vi "Read XML_Parse BC Major Frames.vi"(8 "error in (no error)":errorcluster, 10 "channel in":T1, 11 ".NET Refnum in":refnum<k24>) -> (0 "error out":errorcluster, 2 "channel out":T1, 3 ".NET Refnum out":refnum<k24>)   [LabVIEW 2017, in "Ballard 1553 System Explorer.lvlib"]
uses:
  Ballard 1553 System Explorer.lvlib
  Ballard_Channel.ctl
  Ballard_BC.ctl
  Ballard_message.ctl
  Ballard_messageType.ctl
  Ballard_CWD1.ctl
  Ballard_CWD2.ctl
  Ballard_minorFrame.ctl
  Ballard_majorFrame.ctl
  Ballard_acyclicFrame.ctl
  Ballard_RT.ctl
  Ballard_RT subAddress.ctl
  Ballard_RT direction.ctl
  Ballard_RT rtMode.ctl
  Ballard_RT modeCode.ctl
  D:/Ballard-1553-Custom-Device Inline Async/Source/System Explorer/SubVIs/Parse XML Ballard/Ballard_BTI_XML_MIL_STD_1553_Deserializer.dll
  Ballard_BTI_XML_MIL_STD_1553_Deserializer.dll
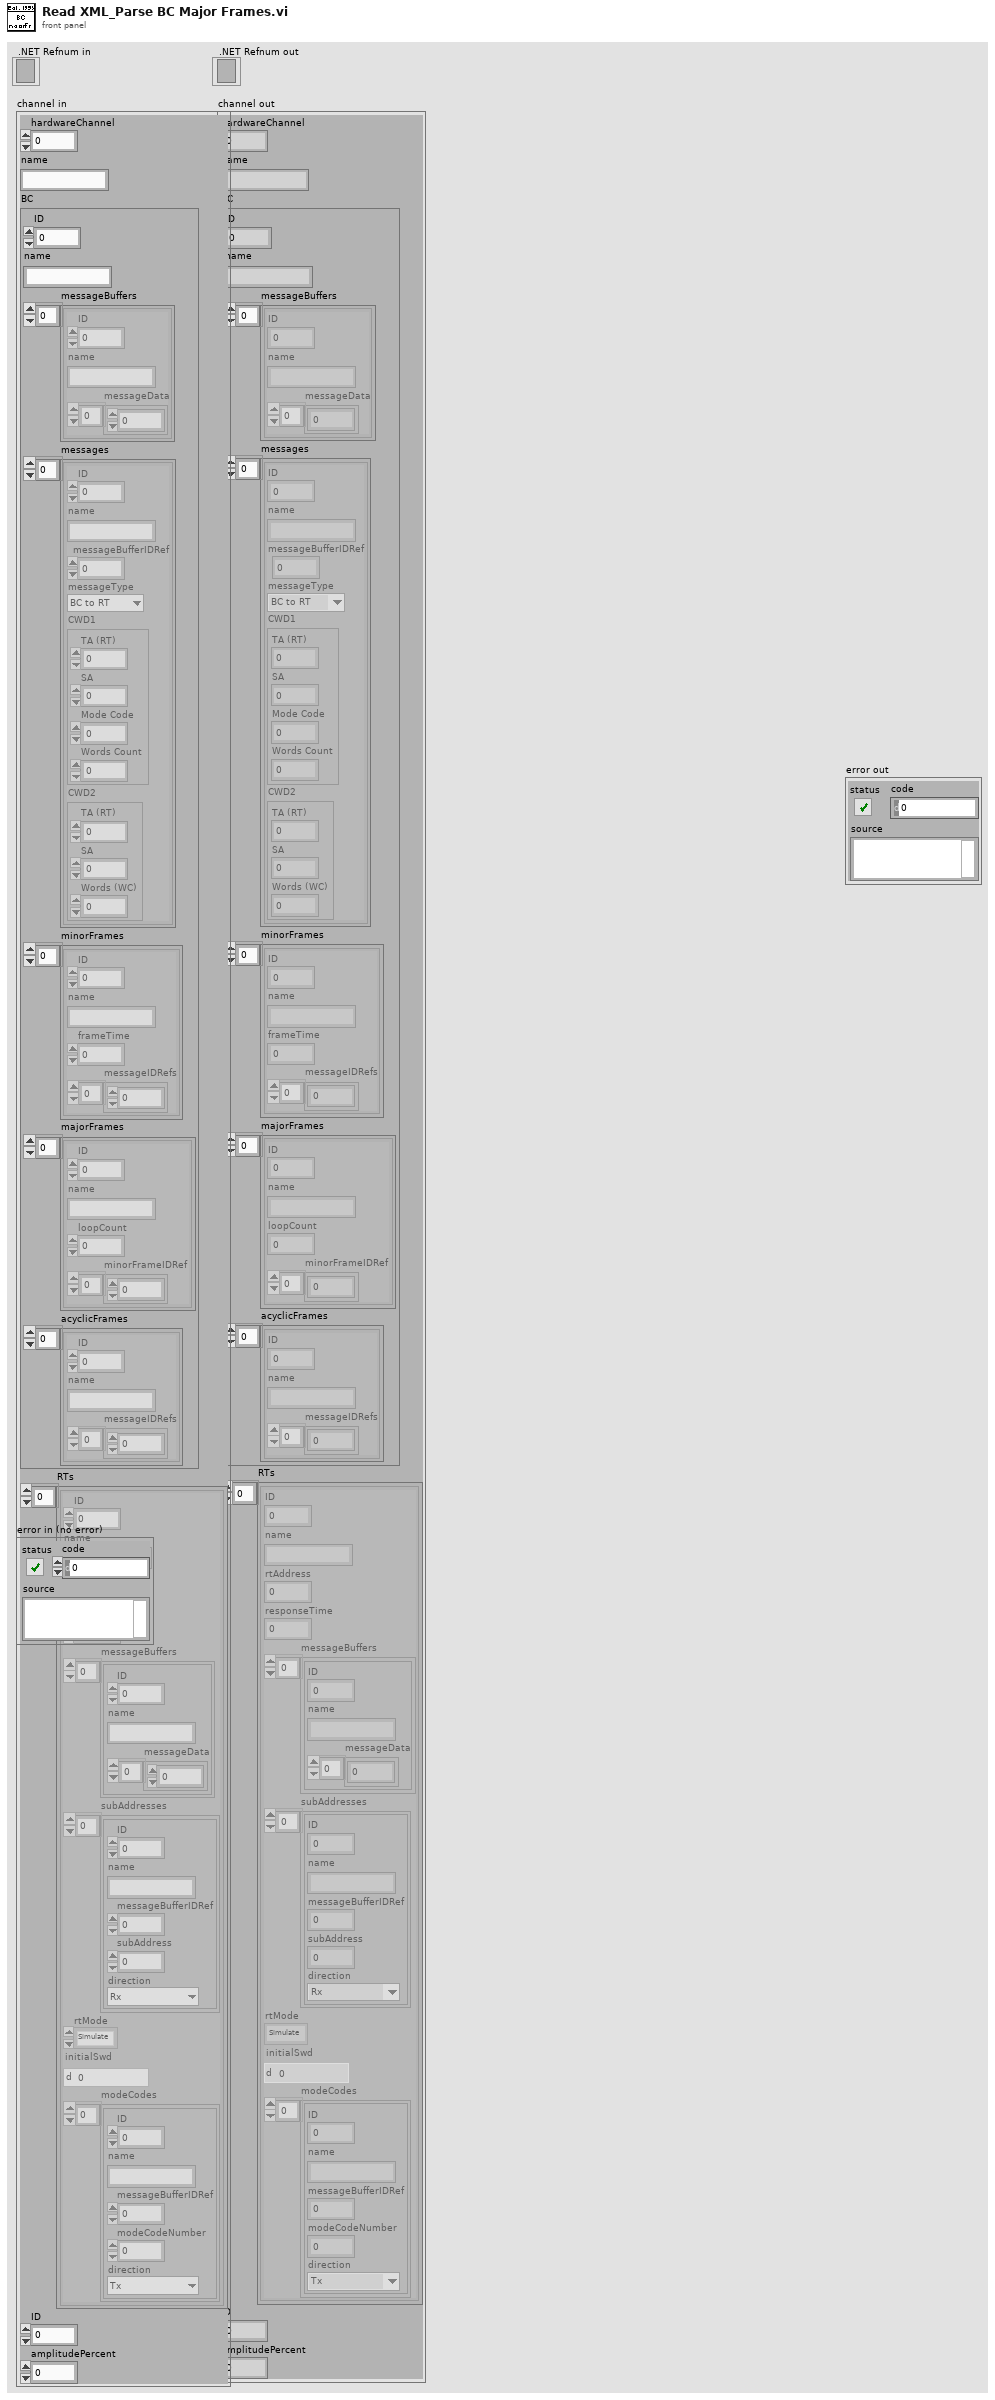
[diagram p1: front panel]
types:
  T1 = typedef "Ballard 1553 System Explorer.lvlib/Ballard_Channel.ctl" = cluster{"hardwareChannel":i32, "name":string, "BC":T2, "RTs":T10[], "ID":i32, "amplitudePercent":dbl}
  T2 = typedef "Ballard 1553 System Explorer.lvlib/Ballard_BC.ctl" = cluster{"ID":i32, "name":string, "messageBuffers":cluster{"ID":i32, "name":string, "messageData":u16[]}[], "messages":T3[], "minorFrames":T7[], "majorFrames":T8[], "acyclicFrames":T9[]}
  T3 = typedef "Ballard 1553 System Explorer.lvlib/Ballard_message.ctl" = cluster{"ID":i32, "name":string, "messageBufferIDRef":i32, "messageType":T4, "CWD1":T5, "CWD2":T6}
  T4 = typedef "Ballard 1553 System Explorer.lvlib/Ballard_messageType.ctl" = enum16{"BC to RT", "RT to BC", "RT to RT", "MC (Rx)", "MC (Tx)"}
  T5 = typedef "Ballard 1553 System Explorer.lvlib/Ballard_CWD1.ctl" = cluster{"TA (RT)":i8, "SA":i8, "Mode Code":i8, "Words Count":i8}
  T6 = typedef "Ballard 1553 System Explorer.lvlib/Ballard_CWD2.ctl" = cluster{"TA (RT)":i8, "SA":i8, "Words (WC)":i8}
  T7 = typedef "Ballard 1553 System Explorer.lvlib/Ballard_minorFrame.ctl" = cluster{"ID":i32, "name":string, "frameTime":i32, "messageIDRefs":i32[]}
  T8 = typedef "Ballard 1553 System Explorer.lvlib/Ballard_majorFrame.ctl" = cluster{"ID":i32, "name":string, "loopCount":i32, "minorFrameIDRef":i32[]}
  T9 = typedef "Ballard 1553 System Explorer.lvlib/Ballard_acyclicFrame.ctl" = cluster{"ID":i32, "name":string, "messageIDRefs":i32[]}
  T10 = typedef "Ballard 1553 System Explorer.lvlib/Ballard_RT.ctl" = cluster{"ID":i32, "name":string, "rtAddress":i8, "responseTime":i32, "messageBuffers":cluster{"ID":i32, "name":string, "messageData":u16[]}[], "subAddresses":T11[], "rtMode":T13, "initialSwd":u16, "modeCodes":T14[]}
  T11 = typedef "Ballard 1553 System Explorer.lvlib/Ballard_RT subAddress.ctl" = cluster{"ID":i32, "name":string, "messageBufferIDRef":i32, "subAddress":i8, "direction":T12}
  T12 = typedef "Ballard 1553 System Explorer.lvlib/Ballard_RT direction.ctl" = enum16{"Tx", "Rx"}
  T13 = typedef "Ballard 1553 System Explorer.lvlib/Ballard_RT rtMode.ctl" = enum16{"Simulate", "Monitor", "Disable"}
  T14 = typedef "Ballard 1553 System Explorer.lvlib/Ballard_RT modeCode.ctl" = cluster{"ID":i32, "name":string, "messageBufferIDRef":i32, "modeCodeNumber":i8, "direction":T12}
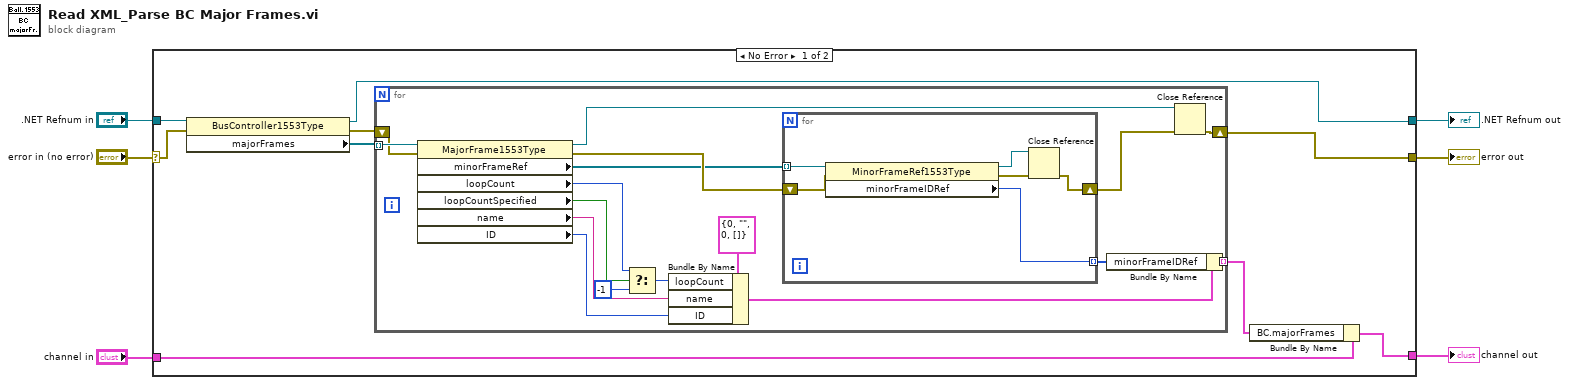
[diagram p0: block diagram]
diagram:
  n1 = case shown="No Error" "error in (no error)" {
    selector: "error in (no error)" -> [w7 w40]
    tunnel: [w14 w39] -> w6
    tunnel: "channel in" -> [w12 w39]
    tunnel: [w10 w41] -> w4
    tunnel: ".NET Refnum in" -> [w9 w41]
    tunnel: [w8 w40] -> w2
    frame No Error {
      n2 = property class="BusController1553Type"(reference=w9, error in=w7) -> (reference out=w10:refnum<k24>, error out=w15:errorcluster, "majorFrames"=w11:refnum<k24>[])
      n3 = for {
        tunnel: w11 -> [w32] mode=indexing
        shift-right: [w29] -> w8
        shift-left: w15 -> [w31]
        tunnel: [w22] -> w13 mode=indexing
        n4 = property class="MajorFrame1553Type"(reference=w32, error in=w31) -> (reference out=w30:refnum<k24>, error out=w26:errorcluster, "minorFrameRef"=w17:refnum<k24>[], "loopCount"=w18:i32, "loopCountSpecified"=w20:bool, "name"=w27:string, "ID"=w28:i32)
        n5 = Select(t=w18, s=w20, f=-1) -> (s? t:f=w21:i32)
        n6 = Bundle By Name(cluster=T8 {"ID"=0, "name"="", "loopCount"=0, "minorFrameIDRef"=[]} ("majorFrame"), "loopCount"=w21, "name"=w27, "ID"=w28) -> (w23:T8)
        n7 = for {
          tunnel: w17 -> [w37] mode=indexing
          shift-right: [w34] -> w25
          shift-left: w26 -> [w38]
          tunnel: [w33] -> w16 mode=indexing
          n8 = property class="MinorFrameRef1553Type"(reference=w37, error in=w38) -> (reference out=w35:refnum<k24>, error out=w36:errorcluster, "minorFrameIDRef"=w33:i32)
          n9 = Close Reference(reference=w35, error in (no error)=w36) -> (error out=w34:errorcluster)
        }
        n10 = Bundle By Name(cluster=w23, "minorFrameIDRef"=w16) -> (w22:T8)
        n11 = Close Reference(reference=w30, error in (no error)=w25) -> (error out=w29:errorcluster)
      }
      n12 = Bundle By Name(cluster=w12, "BC.majorFrames"=w13) -> (w14:T1)
    }
    frame Error {
    }
  }
  "channel out" <- w6
  ".NET Refnum out" <- w4
  "error out" <- w2
